vi "Pre Launch Init.vi"(11 "DAQ Actor in":refnum<class "DAQ Actor.lvclass">) -> (0 "error out":errorcluster, 3 "DAQ Actor out":refnum<class "DAQ Actor.lvclass">)   [LabVIEW 2012, in "Data Acquisition.lvlib" / "DAQ Actor.lvclass"]
doc: "(<B>Filename</B>: Actor Framework.lvlib:Actor.lvclass:Pre Launch Init.vi)\n\nDefines behavior that occurs after the Launch Actor method is invoked but before the actor's Actor Core method begins running.\n\nThe Pre Launch Init method is guaranteed to finish before the Launch Actor method returns to its caller and before the actor itself receives any messages. Any references that the Pre Launch Init method obtains are guaranteed to have the same lifetime as the actor itself. Any errors that the Pre Launch Init method returns will abort the launch.\n\nBy default, this method does nothing. A descendant class may override it to define behavior."
uses:
  DAQ Actor.lvclass
  <vilib>/ActorFramework/Actor/Actor.lvclass
  DAQ Actor.lvclass/DAQ Actor.ctl
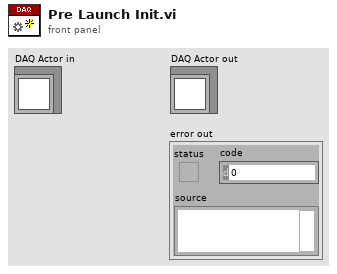
[diagram p1: front panel]
types:
  T1 = typedef "TE_Designator.ctl" = enum16{"High Speed", "Low Speed"}
  T2 = enum16{"Read", "Write", "ReadWrite", "BufferedRead", "BufferedReadWrite"}
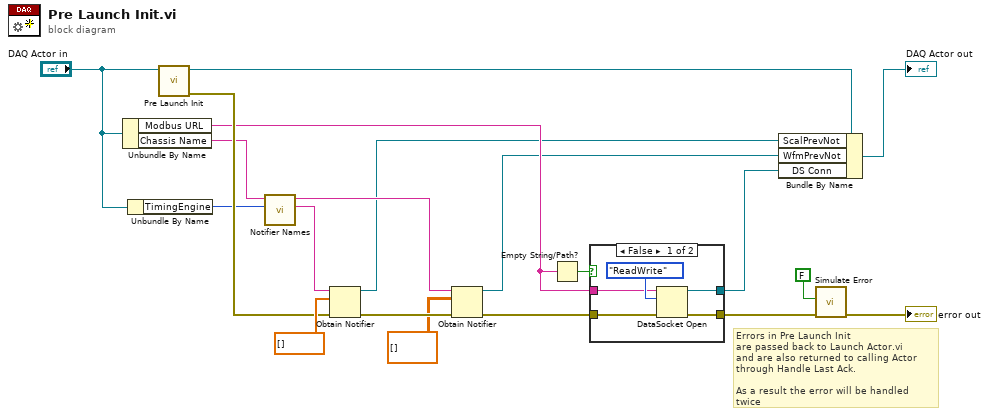
[diagram p0: block diagram]
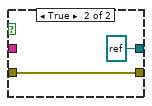
[diagram p2: hidden frame]
diagram:
  # "Errors in Pre Launch Init\nare passed back to Launch Actor.vi\nand are also returned to calling Actor\nthrough Handle Last Ack.\n\nAs a result the error will be handled twice"
  n1 = Unbundle By Name("DAQ Actor in") -> ("Modbus URL"=w9:string, "Chassis Name"=w11:string)
  n2 = Unbundle By Name("DAQ Actor in") -> ("TimingEngine"=w13:T1)
  n3 = call-parent "Pre Launch Init.vi"("Actor in"="DAQ Actor in") -> ("error out"=w14:errorcluster, "Actor out"=w10:refnum<class "DAQ Actor.lvclass">)  [unwired: 9 in]
  n4 = call "Notifier Names.vi"("TimingEngine"=w13, "Chassis Name"=w11) -> ("Scalar Notifier"=w18:string, "Wfm Notifier"=w17:string)  [unwired: 8 in]
  n5 = Obtain Notifier(name (unnamed)=w18, notification data type=dbl[] [], error in (no error)=w14) -> (notifier out=w8:refnum<notifier>, error out=w20:errorcluster)  [unwired: 1 in, 1 out]
  n6 = Obtain Notifier(name (unnamed)=w17, notification data type=dbl[][] [], error in (no error)=w20) -> (notifier out=w1:refnum<notifier>, error out=w15:errorcluster)  [unwired: 1 in, 1 out]
  n7 = Empty String/Path?(string/path=w9) -> (empty?=w16:bool)
  n8 = case shown="False" w16 {
    tunnel: w15 -> [w24 w27]
    tunnel: [w23 w27] -> w4
    tunnel: w9 -> [w22 _]
    tunnel: [w21 refnum<k13> refnum ("connection id")] -> w7
    frame False {
      n9 = DataSocket Open(8:w24, 10:T2."ReadWrite" ("mode"), 11:w22) -> (0:w23:errorcluster, 3:w21:refnum<k13>)  [unwired: 1 in]
    }
    frame True {
    }
  }
  n10 = Bundle By Name(cluster=w10, "ScalPrevNot"=w8, "WfmPrevNot"=w1, "DS Conn"=w7) -> (→"DAQ Actor out":refnum<class "DAQ Actor.lvclass">)
  n11 = call "Simulate Error.vi"("error in (no error)"=w4, "Sim Error?"=FALSE) -> ("error out"=→"error out":errorcluster)  [unwired: 9 in]
